vi "SPI Write Read N Frames.vi"(5 "CS Configuration":T1, 7 "SPI Channel (0)":u8, 8 "Error In":errorcluster, 9 "SPI Frame Size (0)":u8, 10 "Data":u8[](array[numeric]), 11 "LINX Resource":T3) -> (0 "Error Out":errorcluster, 2 "Read Data":u8[](array[numeric]), 3 "LINX Resource":T3)   [LabVIEW 2014, in "LMH-LINX.lvlib"]
doc: "Transmit data on the specified SPI channel and read the response. This VI breaks the transmission up into multiple frames where each frame consists of setting CS active, shifting out a subset of the data bytes, then setting CS idle.\n\nSPI is full duplex, therefore the write and read operations take place simultaneously.\n\n<b>SPI Channel</b> specifies the SPI channel to write/read to.\n\n<b>Data</b> is a U8 array of data bytes to shift out starting with Data[0] to Data[n-1].\n\n<b>SPI Frame Size</b> specifies the number of bytes shifted out between toggling CS.\n\n<b>CS Channel</b> specifies the Chip Select (DIO) channel to use during the SPI transaction.\n\n<b>CS Logic Level</b> specifies the polarity of the chip select output. Active low is most common and results in CS starting in the idle/high state and data being trasnmitted after CS is driven to the active/low state."
uses:
  LMH-LINX.lvlib
  Private/Type Defs/LINX Ref.ctl
  Private/Type Defs/Platform.ctl
  Private/Type Defs/Interface.ctl
  Private/Device/Type Defs/LINX Device Config.ctl
  Private/Device/Type Defs/TCP Config.ctl
  Private/Device/Type Defs/Channels.ctl
  SPI CS Config.ctl
  Private/Type Defs/Peripherals/SPI/SPI CS Logic Level.ctl
  Private/Type Defs/Peripheral.ctl
  Private/Type Defs/Channel FGV States.ctl
  <vilib>/myRIO/Instrument Drivers/Onboard IO/SPI/typedefs/SPI Reference.ctl
  <vilib>/myRIO/Common/Instrument Driver Framework/Utilities/typedefs/myRIO Generic Hardware Reference.ctl
  <vilib>/myRIO/Common/Instrument Driver Framework/Utilities/typedefs/Hardware Version Enum.ctl
  <vilib>/myRIO/Common/Instrument Driver Framework/Utilities/typedefs/myRIO v1.0 Reference.ctl
  <vilib>/myRIO/Common/Instrument Driver Framework/Utilities/typedefs/Generic FPGA Reference.ctl
  <vilib>/myRIO/Common/Instrument Driver Framework/myRIO v1.0/SPI/typedefs/SPI Channels Enum.ctl
  <vilib>/myRIO/Instrument Drivers/Onboard IO/SPI/typedefs/SPI Configuration.ctl
  <vilib>/myRIO/Common/Instrument Driver Framework/myRIO v1.0/SPI/typedefs/SPI Clock Phase.ctl
  <vilib>/myRIO/Common/Instrument Driver Framework/myRIO v1.0/SPI/typedefs/SPI Clock Polarity.ctl
  <vilib>/myRIO/Common/Instrument Driver Framework/myRIO v1.0/SPI/typedefs/SPI Data Direction.ctl
  <vilib>/myRIO/Common/Instrument Driver Framework/myRIO v1.0/SPI/typedefs/SPI Frame Length.ctl
  Private/Device/Device.lvlib
  <vilib>/myRIO/Instrument Drivers/Onboard IO/SPI/SPI.lvlib
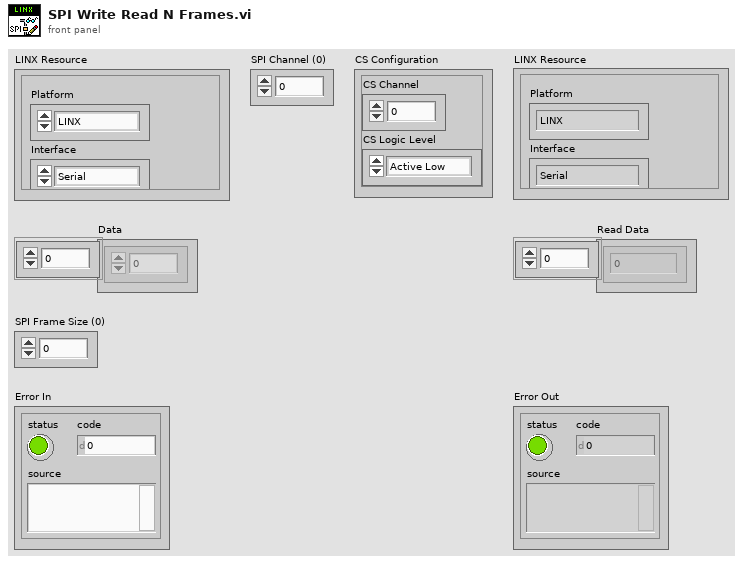
[diagram p1: front panel]
types:
  T1 = typedef "LMH-LINX.lvlib/SPI CS Config.ctl" = cluster{"CS Channel":u8, "CS Logic Level":T2}
  T2 = typedef "LMH-LINX.lvlib/SPI CS Logic Level.ctl" = enum8{"Active Low", "Active High"}
  T3 = typedef "LMH-LINX.lvlib/LINX Ref.ctl" = cluster{"Platform":T4, "Interface":T5, "LINX Device Config":T6}
  T4 = typedef "LMH-LINX.lvlib/Platform.ctl" = enum16{"LINX", "myRIO"}
  T5 = typedef "LMH-LINX.lvlib/Interface.ctl" = enum16{"Serial", "TCP"}
  T6 = typedef "LMH-LINX.lvlib/Device.lvlib/LINX Device Config.ctl" = cluster{"Interface":T5, "COM Port":refnum<visa-resource-name>, "TCP Configuration":T7, "Device Family":u8, "Device ID":u8, "Device Name":string, "TCP Ref":refnum<k5>, "Channels":T8}
  T7 = typedef "LMH-LINX.lvlib/Device.lvlib/TCP Config.ctl" = cluster{"IP Address":string, "Port":u16}
  T8 = typedef "LMH-LINX.lvlib/Channels.ctl" = cluster{"DI":u8[], "DO":u8[], "AI":u8[], "AO":u8[], "PWM":u8[], "QE":u8[], "UART":u8[], "I2C 2":u8[], "SPI":u8[], "CAN":u8[], "Servo":u8[], "AI Ref (V)":dbl, "AO Ref (V)":dbl, "AO Resolution (Bits)":u8}
  T9 = typedef "LMH-LINX.lvlib/Peripheral.ctl" = enum8{"DI", "DO", "AI", "AO", "PWM", "QE", "UART", "I2C", "SPI", "CAN", "Servo"}
  T10 = typedef "LMH-LINX.lvlib/Channel FGV States.ctl" = enum16{"Initialize", "Get", "Set"}
  T11 = typedef "SPI.lvlib/SPI Reference.ctl" = cluster{"myRIO Reference":T12, "SPI Channels Enum":T16, "SPI Configuration":T17}
  T12 = typedef "myRIO Generic Hardware Reference.ctl" = cluster{"myRIO Model":T13, "myRIO Hardware Reference":T14}
  T13 = typedef "Hardware Version Enum.ctl" = enum16{"Unknown", "myRIO-1900", "myRIO-1950"}
  T14 = typedef "myRIO v1.0 Reference.ctl" = cluster{"Generic FPGA Reference":T15, "Allow multiple opens":bool}
  T15 = typedef "Generic FPGA Reference.ctl" = refnum<k20>
  T16 = typedef "SPI Channels Enum.ctl" = enum16{"Not Connected", "A/SPI", "B/SPI"}
  T17 = typedef "SPI.lvlib/SPI Configuration.ctl" = cluster{"Frequency [Hz]":dbl, "Clock Phase":T18, "Clock Polarity":T19, "Data Direction":T20, "Frame Length":T21}
  T18 = typedef "SPI Clock Phase.ctl" = enum8{"Leading", "Trailing"}
  T19 = typedef "SPI Clock Polarity.ctl" = enum8{"Low", "High"}
  T20 = typedef "SPI Data Direction.ctl" = enum8{"Most significant bit first", "Least significant bit first"}
  T21 = typedef "SPI Frame Length.ctl" = u8
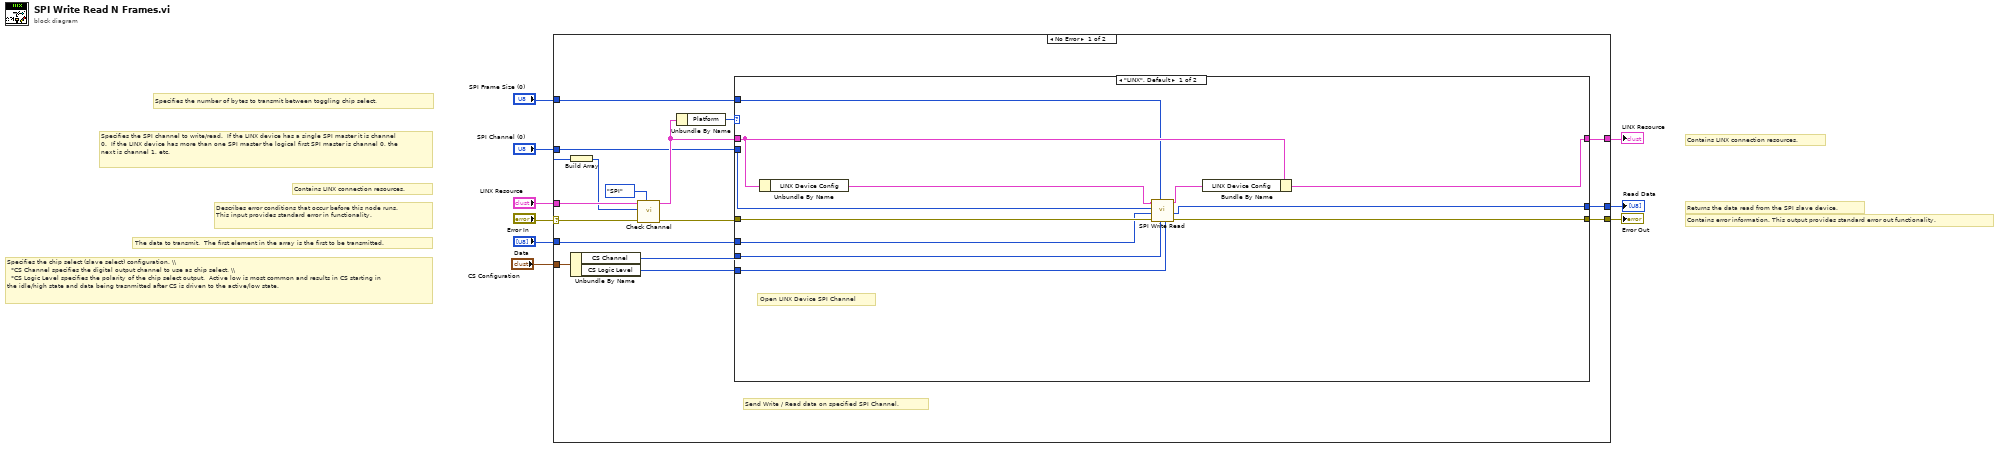
[diagram p0: block diagram]
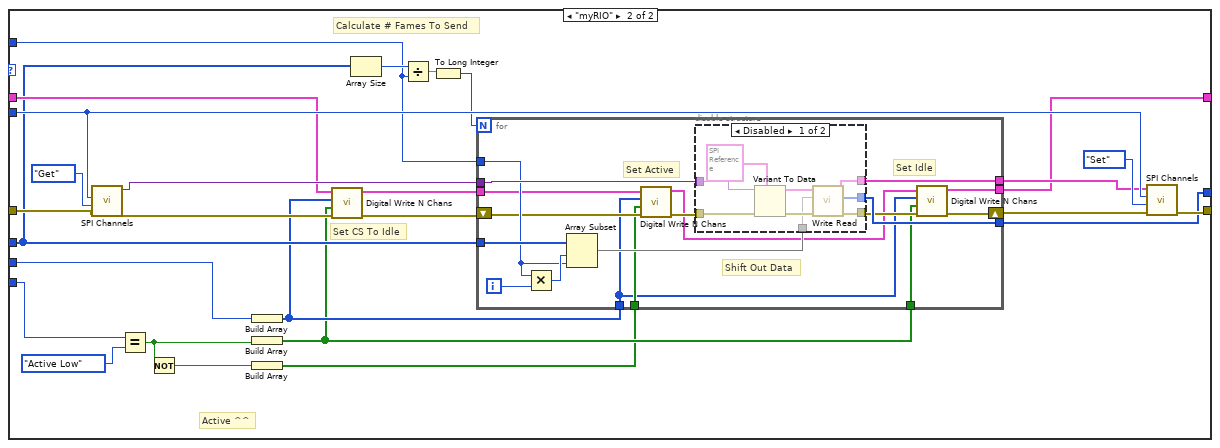
[diagram p2: hidden frame]
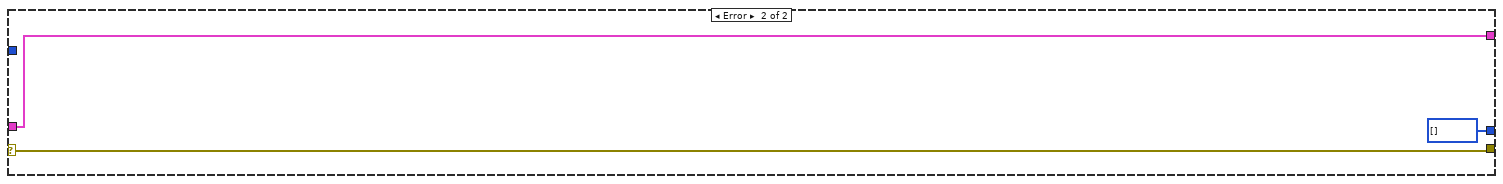
[diagram p4: hidden frame]
diagram:
  # "Returns the data read from the SPI slave device."
  # "Contains error information. This output provides standard error out functionality."
  # "Specifies the chip select (slave select) configuration. \\\\\n  *CS Channel specifies the digital output channel to use as chip select. \\\\ \n  *CS Logic Level specifies the polarity of the chip select output.  Active low is most common and results in CS starting in the idle/high state and data being trasnmitted after CS is driven to the active/low state."
  # "Specifies the number of bytes to transmit between toggling chip select."
  # "The data to transmit.  The first element in the array is the first to be transmitted."
  # "Specifies the SPI channel to write/read.  If the LINX device has a single SPI master it is channel 0.  If the LINX device has more than one SPI master the logical first SPI master is channel 0, the next is channel 1, etc."
  # "Contains LINX connection resources."
  # "Contains LINX connection resources."
  # "Describes error conditions that occur before this node runs. This input provides standard error in functionality."
  n1 = case shown="No Error" "Error In" {
    selector: "Error In" -> [w10 w94]
    tunnel: [w24 w94] -> w9
    tunnel: "LINX Resource" -> [w23 w92]
    tunnel: "SPI Channel (0)" -> [w19 _]
    tunnel: [w17 u16[] [] ("Frames Read")] -> w6
    tunnel: "Data" -> [w16 _]
    tunnel: "SPI Frame Size (0)" -> [w15 _]
    tunnel: [w14 w92] -> w3
    tunnel: "CS Configuration" -> [w13 _]
    frame No Error {
      # "Send Write / Read data on specified SPI Channel."
      n2 = Unbundle By Name(w13) -> ("CS Channel"=w12:u8, "CS Logic Level"=w11:T2)
      n3 = Build Array(w19) -> (w20:u8[])
      n4 = call "Check Channel.vi"("Peripheral"=Peripheral."SPI", "Error In"=w10, "Channels"=w20, "LINX Resource"=w23) -> ("Error Out"=w21:errorcluster, "LINX Resource"=w22:T3)  [unwired: 5 in, 1 out]
      n5 = Unbundle By Name(w22) -> ("Platform"=w25:T4)
      n6 = case shown="\"LINX\", Default" w25 {
        tunnel: w21 -> [w35 w62]
        tunnel: w22 -> [w37 w55]
        tunnel: [w36 w64] -> w24
        tunnel: [w26 w43] -> w14
        tunnel: w19 -> [w30 w61]
        tunnel: [w32 w56] -> w17
        tunnel: w16 -> [w31 w50]
        tunnel: w15 -> [w29 w46]
        tunnel: w12 -> [w28 w42]
        tunnel: w11 -> [w27 w52]
        frame "LINX", Default {
          # "Open LINX Device SPI Channel"
          n7 = Unbundle By Name(w37) -> ("LINX Device Config"=w33:T6)
          n8 = call "SPI Write Read.vi"("CS Logic Level"=w27, "CS Pin (10)"=w28, "SPI Frame Size (1)"=w29, "Error In"=w35, "Data"=w31, "SPI Channel"=w30, "LINX Device Config"=w33) -> ("Error Out"=w36:errorcluster, "Read Data"=w32:u8[], "LINX Device Config"=w34:T6)  [unwired: 2 in]
          n9 = Bundle By Name(cluster=w37, "LINX Device Config"=w34) -> (w26:T3)
        }
        frame "myRIO" {
          # "Active ^^"
          # "Calculate # Fames To Send"
          # "Set CS To Idle"
          n10 = call "SPI Channels.vi"("Error In"=w62, "Channel State"=Channel_FGV_States."Get", "Channel Number"=w61) -> ("Error Out"=w54:errorcluster, "SPI Channel"=w57:variant)  [unwired: 7 in]
          n11 = Equal?(x=w52, y=SPI_CS_Logic_Level."Active Low") -> (x = y?=w41:bool)
          n12 = Not(x=w41) -> (.not. x?=w39:bool)
          n13 = Build Array(w42) -> (w44:u8[])
          n14 = Build Array(w41) -> (w40:bool[])
          n15 = Build Array(w39) -> (w38:bool[])
          n16 = call "Digital Write N Chans.vi"("Error In"=w54, "Values"=w40, "DO Channels"=w44, "LINX Resource"=w55) -> ("Error Out"=w53:errorcluster, "LINX Resource"=w45:T3)  [unwired: 6 in]
          n17 = Array Size(array=w50) -> (size(s)=w49:i32)
          n18 = Divide(x=w49, y=w46) -> (x/y=w48:dbl)
          n19 = To Long Integer(number=w48) -> (32bit integer=w47:i32)
          n20 = for {
            N: w47 -> [_]
            tunnel: [w82] -> w58
            tunnel: w57 -> [w81]
            tunnel: w50 -> [w79]
            tunnel: [w80] -> w56
            shift-right: [w71] -> w59
            shift-left: w53 -> [w74]
            tunnel: w46 -> [w75]
            tunnel: w45 -> [w72]
            tunnel: w44 -> [w65]
            tunnel: [w68] -> w43
            tunnel: w40 -> [w67]
            tunnel: w38 -> [w66]
            i -> [w77]
            # "Set Idle"
            # "Shift Out Data"
            # "Set Active"
            n21 = Multiply(x=w75, y=w77) -> (x*y=w76:i32)
            n22 = Array Subset(array=w79, index=w76, length=w75) -> (w78:u8[])
            n23 = call "Digital Write N Chans.vi"("Error In"=w74, "Values"=w66, "DO Channels"=w65, "LINX Resource"=w72) -> ("Error Out"=w73:errorcluster, "LINX Resource"=w69:T3)  [unwired: 6 in]
            n24 = disable-structure shown="Disabled" {
              disable-tunnel: [w89 _] -> w70
              disable-tunnel: w73 -> [w87 _]
              disable-tunnel: [w86 _] -> w82
              disable-tunnel: w81 -> [w85 _]
              disable-tunnel: w78 -> [w84 _]
              disable-tunnel: [w83 _] -> w80
              frame Disabled {
                n25 = Variant To Data(error in=w87, type=T11 {"myRIO Reference"={"myRIO Model"=enum."Unknown", "myRIO Hardware Reference"={"Generic FPGA Reference"=refnum, "Allow multiple opens"=FALSE}}, "SPI Channels Enum"=enum."Not Connected", "SPI Configuration"={"Frequency [Hz]"=0.0, "Clock Phase"=enum."Leading", "Clock Polarity"=enum."Low", "Data Direction"=enum."Most significant bit first", "Frame Length"=8}} ("SPI Ref In"), Variant=w85) -> (data=w90:T11, error out=w88:errorcluster)
                n26 = call <vilib>:"Write Read.vi"("error in (no error)"=w88, "Frames to Write"=w84, "SPI Ref In"=w90) -> ("error out"=w89:errorcluster, "Frames Read"=w83:u16[], "SPI Ref Out"=w86:T11)  [unwired: 6 in]
              }
              frame Enabled {
              }
            }
            n27 = call "Digital Write N Chans.vi"("Error In"=w70, "Values"=w67, "DO Channels"=w65, "LINX Resource"=w69) -> ("Error Out"=w71:errorcluster, "LINX Resource"=w68:T3)  [unwired: 6 in]
          }
          n28 = call "SPI Channels.vi"("Error In"=w59, "Channel State"=Channel_FGV_States."Set", "Channel Number"=w61, "SPI Channel"=w58) -> ("Error Out"=w64:errorcluster)  [unwired: 6 in, 1 out]
        }
      }
    }
    frame Error {
    }
  }
  "Error Out" <- w9
  "LINX Resource" <- w3
  "Read Data" <- w6
